vi "Count up U8.vi"(8 "reset":bool=TRUE, 10 "increment":bool=TRUE) -> (2 "count out":u8)   [LabVIEW 2020]
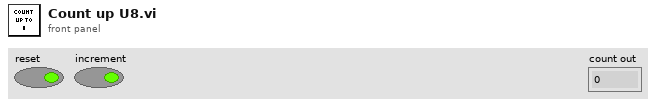
[diagram p1: front panel]
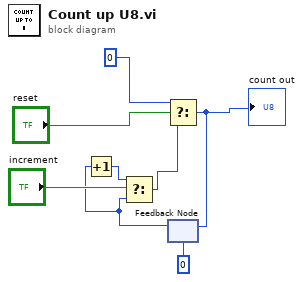
[diagram p0: block diagram]
diagram:
  n1 = feedback #1(u8 0) -> (w1:u8)
  n2 = Increment(x=w1) -> (x+1=w2:u8)
  n3 = Select(t=w2, s="increment", f=w1) -> (s? t:f=w5:u8)
  n4 = Select(t=u8 0, s="reset", f=w5) -> (s? t:f=w4:u8)
  "count out" <- w4
  n5 = feedback-in #1(w4) -> ()
